vi "Approximately equals (DBL).vi"(7 "dy":dbl, 10 "y":dbl, 11 "x":dbl) -> (3 "x between (y-dy),(y+dy)?":bool)   [LabVIEW 2014, in "COSYLib.lvlib"]
doc: "Returns TRUE if x falls within the range (y-dy, y+dy)."
uses:
  COSYLib.lvlib
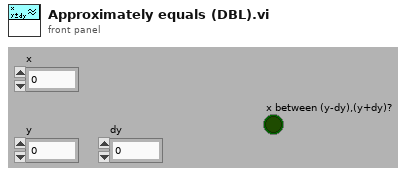
[diagram p1: front panel]
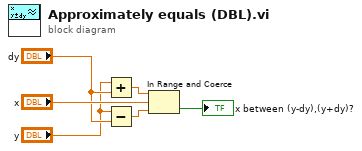
[diagram p0: block diagram]
diagram:
  n1 = Add(x="y", y="dy") -> (x+y=w3:dbl)
  n2 = Subtract(x="y", y="dy") -> (x-y=w4:dbl)
  n3 = In Range and Coerce(upper limit=w3, x="x", lower limit=w4) -> (In Range?=→"x between (y-dy),(y+dy)?":bool)  [unwired: 1 out]
